vi "Remove_Tag.vi"(8 "error in":errorcluster, 10 "tag":string, 11 "Tree Refnum":refnum<vi>) -> (0 "error out":errorcluster, 3 "selected tag":string)   [LabVIEW 2020, in "IB_Tree.lvclass"]
uses:
  <vilib>/AppBuilder/IB_Classes/Tree/IB_Tree.lvclass
  <vilib>/AppBuilder/IB_Classes/Tree/IB_Tree.lvclass/IB_Tree.ctl
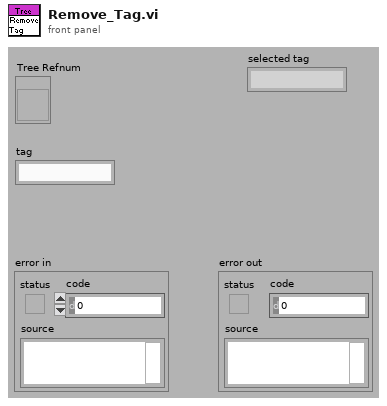
[diagram p1: front panel]
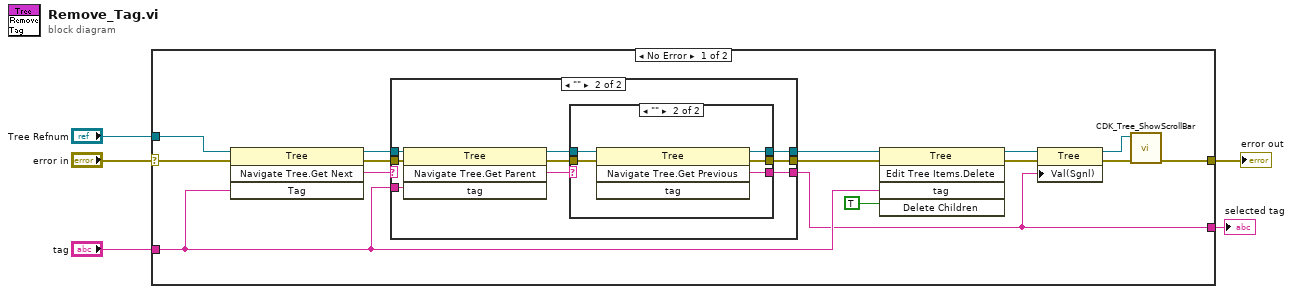
[diagram p0: block diagram]
diagram:
  n1 = case shown="No Error" "error in" {
    selector: "error in" -> [w7 w41]
    tunnel: "tag" -> [w19 _]
    tunnel: "Tree Refnum" -> [w18 _]
    tunnel: [w9 w41] -> w3
    tunnel: [w6 _] -> w1
    frame No Error {
      n2 = invoke class="Tree" method="Navigate Tree.Get Next"(reference=w18, error in=w7, "Tag"=w19) -> (reference out=w14:refnum<vi>, error out=w16:errorcluster, "Navigate Tree:Get Next Item"=w15:string)  [unwired: 1 in, 1 out]
      n3 = case shown="\"\"" w15 {
        selector: w15 -> [w22 _]
        tunnel: [w22 w24] -> w6
        tunnel: [w21 w25] -> w17
        tunnel: w14 -> [w23 w32]
        tunnel: [w23 w26] -> w20
        tunnel: w19 -> [_ w31]
        tunnel: w16 -> [w21 w30]
        frame Default {
        }
        frame "" {
          n4 = invoke class="Tree" method="Navigate Tree.Get Parent"(reference=w32, error in=w30, "tag"=w31) -> (reference out=w27:refnum<vi>, error out=w28:errorcluster, "Navigate Tree:Get Parent"=w29:string)  [unwired: 1 in, 1 out]
          n5 = case shown="\"\"" w29 {
            selector: w29 -> [w35 _]
            tunnel: w28 -> [w33 w40]
            tunnel: w27 -> [w34 w39]
            tunnel: [w34 w38] -> w26
            tunnel: [w33 w37] -> w25
            tunnel: [w35 w36] -> w24
            frame Default {
            }
            frame "" {
              n6 = invoke class="Tree" method="Navigate Tree.Get Previous"(reference=w39, error in=w40) -> (reference out=w38:refnum<vi>, error out=w37:errorcluster, "Navigate Tree:Get Previous"=w36:string)  [unwired: 2 in, 1 out]
            }
          }
        }
      }
      n7 = invoke class="Tree" method="Edit Tree Items.Delete"(reference=w20, error in=w17, "tag"=w19, "Delete Children"=TRUE ("Delete Children?")) -> (reference out=w10:refnum<vi>, error out=w12:errorcluster)  [unwired: 1 in, 3 out]
      n8 = property class="Tree"(reference=w10, error in=w12, "Val(Sgnl)"=w6) -> (reference out=w11:refnum<vi>, error out=w13:errorcluster)
      n9 = call <resource>:"CDK_Tree_ShowScrollBar.vi"("error in (no error)"=w13, "Tree"=w11) -> ("error out"=w9:errorcluster)  [unwired: 9 in]
    }
    frame Error {
    }
  }
  "error out" <- w3
  "selected tag" <- w1
